vi "ni5660 Close.vi"(0 "receiver info in":T1, 11 "error in (no error)":errorcluster) -> (15 "error out":errorcluster)   [LabVIEW 2011]
doc: "This VI performs the following actions: \n\nAborts any signal acquisition in progress. \nTerminates the instrument I/O session. \nDestroys the instrument driver session and any attributes. \nCall this VI to end every session with the ni5660 VIs."
uses:
  <vilib>/addons/Modulation/niScope/controls/mod_Modulation Settings.ctl
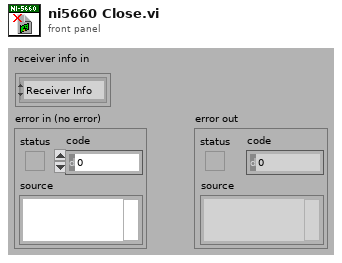
[diagram p1: front panel]
types:
  T1 = typedef "mod_Modulation Settings.ctl" = cluster{enum16{"Receiver Info"}, variant}
  T2 = typedef "mod_Readable Attributes Cluster.ctl" = cluster{"carrier":cluster{"frequency":dbl}, "receiver":cluster{"handles":cluster{"niTuner taskID":i32, "niScope handle":refnum<k15>}, "RFSA":cluster{"reference level":i32, "RF attenuation":i32}, "data format":enum16{"real", "complex modulated (array)", "complex modulated (interleaved)"}, "auto suppress SW IQ":enum16{"off", "on"}, "IQ sample rate":dbl, "bandwidth":dbl}}
  T3 = cluster{"taskID out":i32, "instrument handle":refnum<k15>}
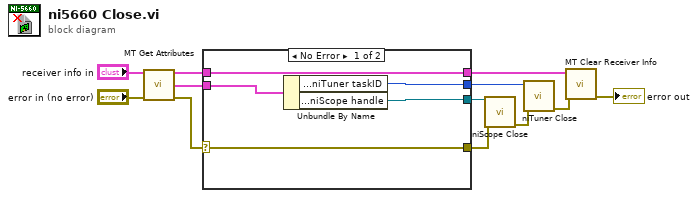
[diagram p0: block diagram]
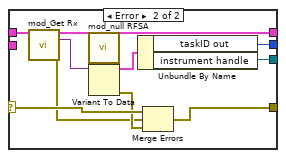
[diagram p2: hidden frame]
diagram:
  n1 = call <vilib>:"MT Get Attributes.vi"("receiver info in"="receiver info in", "error in (no error)"="error in (no error)") -> ("receiver info out"=w5:T1, "attributes"=w7:T2, "error out"=w3:errorcluster)  [unwired: 11 in]
  n2 = case shown="No Error" w3 {
    selector: w3 -> [w16 w23]
    tunnel: w7 -> [w13 _]
    tunnel: [w17 w26] -> w6
    tunnel: w5 -> [w17 w27]
    tunnel: [w16 w21] -> w4
    tunnel: [w15 w20] -> w2
    tunnel: [w14 w19] -> w1
    frame No Error {
      n3 = Unbundle By Name(w13) -> ("receiver.handles.niTuner taskID"=w15:i32, "receiver.handles.niScope handle"=w14:refnum<k15>)
    }
    frame Error {
      n4 = call <vilib>:"mod_Get Rx.vi"("receiver info in"=w27) -> ("receiver info out"=w26:T1, "Rx"=w25:variant, "error out"=w18:errorcluster)  [unwired: 11 in, 1 out]
      n5 = call <vilib>:"mod_null RFSA.vi"() -> ("null RFSA"=w28:T3)
      n6 = Variant To Data(type=w28, Variant=w25) -> (data=w24:T3, error out=w22:errorcluster)  [unwired: 1 in]
      n7 = Unbundle By Name(w24) -> ("taskID out"=w20:i32, "instrument handle"=w19:refnum<k15>)
      n8 = Merge Errors(w23, w18, w22) -> (w21:errorcluster)
    }
  }
  n9 = call <instrlib>:"niScope Close.vi"("instrument handle"=w1, "error in"=w4) -> ("error out"=w11:errorcluster)  [unwired: 13 in]
  n10 = call <instrlib>:"niTuner Close.vi"("error in"=w11, "taskID in"=w2) -> ("error out"=w12:errorcluster)  [unwired: 9 in]
  n11 = call <vilib>:"MT Clear Receiver Info.vi"("receiver info in"=w6, "error in (no error)"=w12) -> ("error out"=→"error out":errorcluster)  [unwired: 13 in]
